vi "Test Missing PPLs.vi"(11 "Test Case In":refnum<class "Missing in Project.lvclass">) -> (0 "error out":errorcluster, 3 "Test Case Out":refnum<class "Missing in Project.lvclass">)   [LabVIEW 2020, in "Missing in Project.lvclass"]
doc: "Tests to make sure all PPLs defined in the project are saved to disk."
uses:
  Missing in Project.lvclass
  C:/Program Files/National Instruments/LabVIEW 2024/vi.lib/Astemes/LUnit/Test Case.lvclass
  <vilib>/Astemes/LUnit/Test Case.lvclass/Test Case.ctl
  <vilib>/Astemes/LUnit/Append Pass Result.vi
  <vilib>/Astemes/LUnit/Append Fail Result.vi
  <vilib>/Astemes/LUnit/Run In UI.vi
  <vilib>/Utility/error.llb/Clear Errors.vi
  <vilib>/Astemes/LUnit/Test Case.lvclass
panel:
  out "Missing items from LabVIEW project":path[](array[path])
  out "Pass":bool
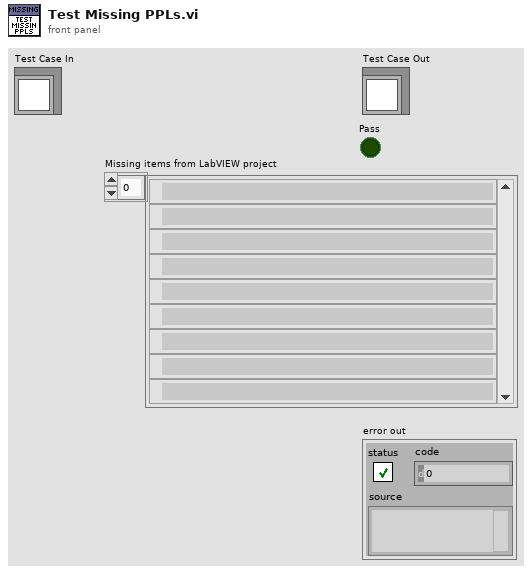
[diagram p1: front panel]
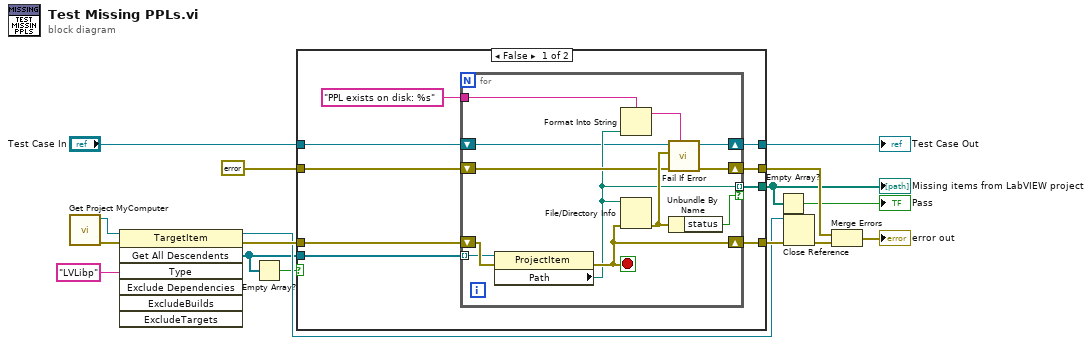
[diagram p0: block diagram]
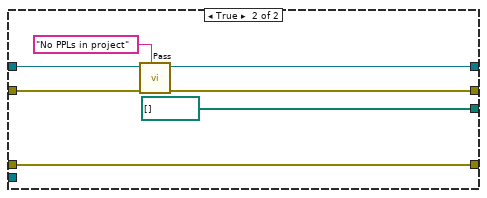
[diagram p2: hidden frame]
diagram:
  n1 = call "Get Project MyComputer.vi"() -> ("error out"=w12:errorcluster, "My Computer"=w5:refnum<vi>)  [unwired: 10 in]
  n2 = invoke class="TargetItem" method="Get All Descendents"(reference=w5, error in=w12, "Type"="LVLibp") -> (reference out=w8:refnum<vi>, error out=w16:errorcluster, "All Descendents"=w2:refnum<vi>[])  [unwired: 4 in, 4 out]
  n3 = Empty Array?(array=w2) -> (empty?=w1:bool)
  n4 = case shown="False" w1 {
    tunnel: w16 -> [w25 w42]
    tunnel: [w24 w42] -> w15
    tunnel: errorcluster {"status"=FALSE, "code"=0, "source"=""} ("error in (no error)") -> [w23 w43]
    tunnel: [w22 w44] -> w11
    tunnel: [w21 path[] []] -> w6
    tunnel: "Test Case In" -> [w19 w40]
    tunnel: [w18 w41] -> w3
    tunnel: w2 -> [w17 _]
    frame False {
      n5 = for {
        tunnel: w17 -> [w32] mode=indexing
        shift-right: [w35] -> w24
        shift-left: w25 -> [w36]
        tunnel: [w31] -> w21 mode=indexing if=w27
        shift-right: [w34] -> w22
        shift-left: w23 -> [w33]
        tunnel: "PPL exists on disk: %s" ("Label") -> [w30]
        shift-right: [w29] -> w18
        shift-left: w19 -> [w28]
        stop <- w35 stop-if-true
        n6 = property class="ProjectItem"(reference=w32, error in=w36) -> (error out=w35:errorcluster, "Path"=w31:path)  [unwired: 1 out]
        n7 = Format Into String(format string=w30, w31) -> (resulting string=w26:string)  [unwired: 2 in, 1 out]
        n8 = File/Directory Info(path=w31, error in=w35) -> (error out=w37:errorcluster)  [unwired: 6 out]
        n9 = call <vilib>:"Fail If Error.vi"("Description"=w26, "error in (no error)"=w33, "Assert error"=w37, "LUnit Test Case In"=w28) -> ("error out"=w34:errorcluster, "LUnit Test Case Out"=w29:refnum<class "Missing in Project.lvclass">)  [unwired: 6 in]
        n10 = Unbundle By Name(w37) -> ("status"=w27:bool)
      }
    }
    frame True {
      n11 = call <vilib>:"Pass.vi"("Description"="No PPLs in project", "error in (no error)"=w43, "LUnit Test Case In"=w40) -> ("error out"=w44:errorcluster, "LUnit Test Case Out"=w41:refnum<class "Missing in Project.lvclass">)  [unwired: 7 in]
    }
  }
  "Missing items from LabVIEW project" <- w6
  "Test Case Out" <- w3
  n12 = Empty Array?(array=w6) -> (empty?=→"Pass":bool)
  n13 = Close Reference(reference=w8, error in (no error)=w15) -> (error out=w14:errorcluster)
  n14 = Merge Errors(w11, w14) -> (→"error out":errorcluster)
